vi "run this file.vi"() -> ()   [LabVIEW 2022 SP3]
uses:
  <vilib>/Platform/TimedLoop/XDataNode/timing_clust.ctl
  <vilib>/Platform/TimedLoop/XDataNode/nitl_modes.ctl
  <vilib>/Platform/TimedLoop/XDataNode/wakeup.ctl
  9477/Public/Configure/Setpoint/Configure Setpoint (Percentage).vi
  9477/Public/Data/Setpoint/Read Setpoint (Direct).vi
  Data/Measure/Read Measure (Direct).vi
  <vilib>/Platform/TimedLoop/XDataNode/XDataNode.xnode
  9477/Bronkhorst FLOW-BUS.lvlib
  <vilib>/Platform/TimedLoop/XDataNode/XDNodeRunTimeDep.lvlib
panel:
  out "Numeric":dbl format="%#_13g"
  out "error out 3":errorcluster
  in  "Path":path
  in  "CH4 setpoint percentage":dbl format="%#_13g"
  in  "Air set point percentage":dbl format="%#_13g"
  in  "CO2 set point percentage":dbl format="%#_13g"
  in  "CH4 Node":i32=5
  in  "Air Node":i32=4
  in  "CO2 Node":i32=18
  in  "VISA resource name":refnum<visa-resource-name>="ASRL2::INSTR"
  in  "Stop":bool=TRUE
  out "error out 2":errorcluster
  out "Unit CH4":string
  out "Setpoint Direct (0) CH4":sgl min=0 step=1 format="%#_5g"
  out "Unit Air":string
  out "Setpoint Direct (0) Air":sgl min=0 step=1 format="%#_5g"
  out "Setpoint Direct (0) CO2":sgl min=0 step=1 format="%#_5g"
  out "Unit CO2":string
  # "#This is the visa input resource address, it depends on which kind of the VISA resource user applying."
  # "#The path is the file path the user woyld like to save."
  # "Time"
  # "CO2 flowrate"
  # "Air flowrate"
  # "CH4 flowrate"
  # "# The node is set by the user on the side of Mass Flow Controller itself, swicth the button to the node address you would like to set. \n# The CO2 MFC was used before, and the CO2 node has been set as 18.\n# The Air and CH4 MFC were not used before, the initial setting of node address is 00. \n These two MFC can only show readings when the node addresses are allocated.\n#The expected flowrate of each MFC is set by the percentage, the capacity can be found on the backside of each MFC.\n#Light the STOP button when the suer wants to stop reading."
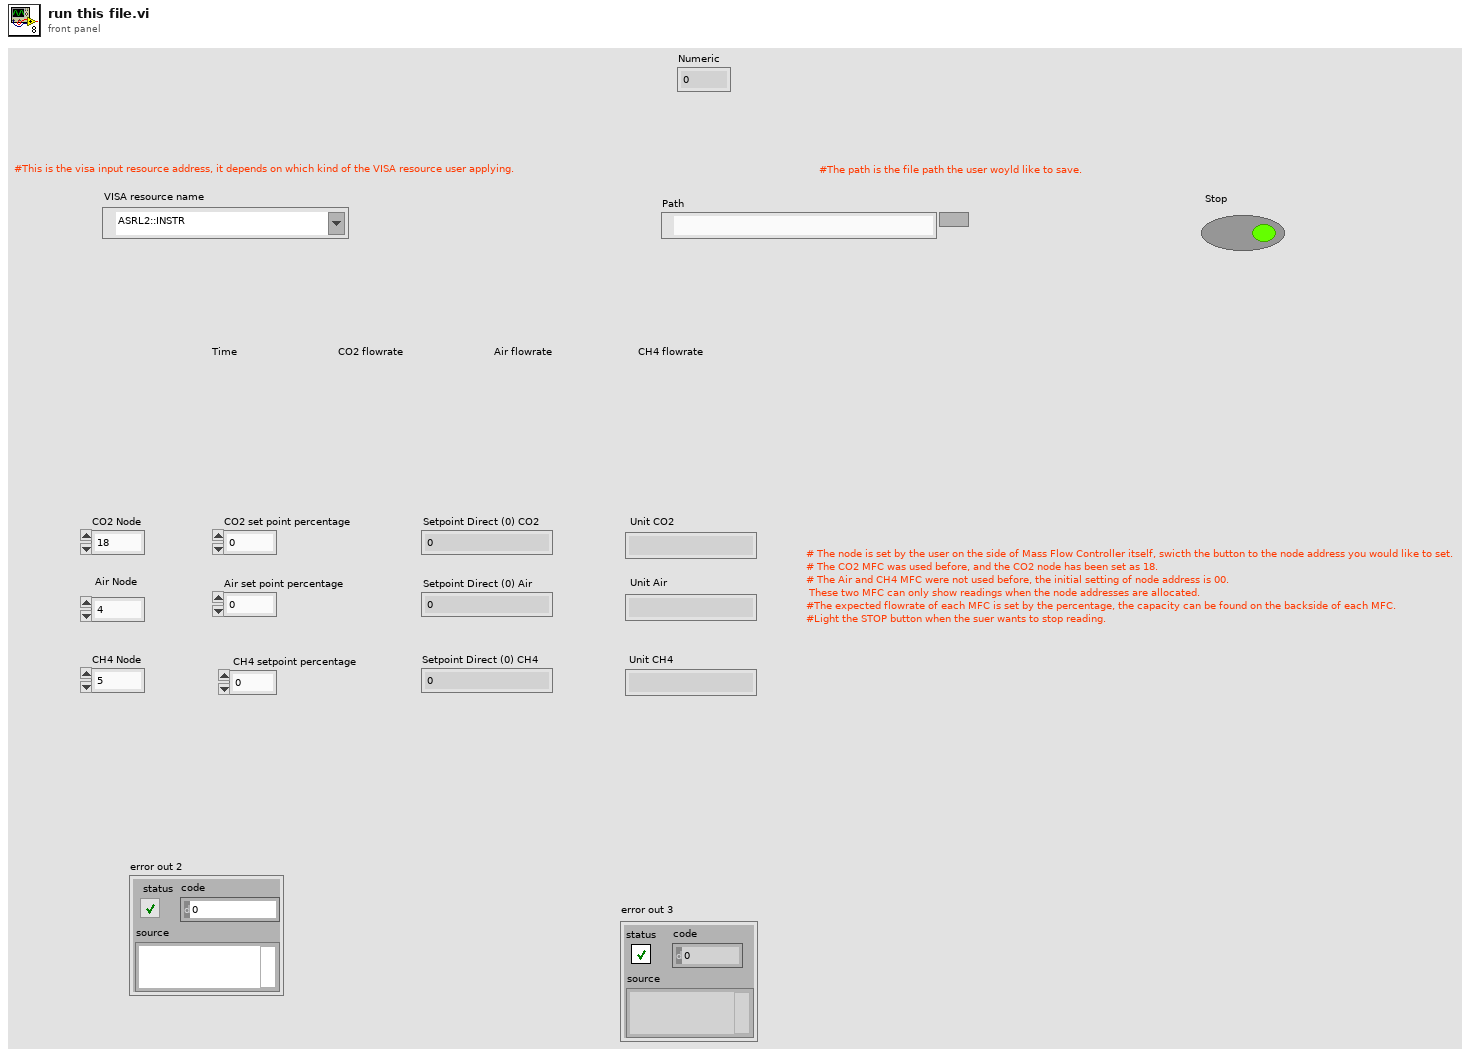
[diagram p1: front panel]
types:
  T1 = enum16{"open", "open or create", "create or replace", "create", "open (read-only)"}
  T2 = typedef "XDNodeRunTimeDep.lvlib/timing_clust.ctl" = cluster{"Expected End [f-1]":u64, "Actual End [f-1]":u64, "Finished Late? [f-1]":bool, "Expected End [i-1]":u64, "Actual End [i-1]":u64, "Finished Late? [i-1]":bool, "Expected Start [i]":u64, "Actual Start [i]":u64, "Expected Start [f]":u64, "Actual Start [f]":u64, "Source Name":string, "Structure Name":string, "Period":i64, "Deadline":i64, "Offset":i64, "Start":i64, "Priority":i32, "Timeout":i32, "Mode":T3, "Wakeup Reason":T4, "Error":errorcluster, "Source Type":string, "Secondary Source Type":string, "Global End Time":u64, "Global Start Time":u64, "Frame Duration":u64, "Iteration Duration":u64, "Assigned CPU":i32, "I/O Scan Engine Mode":u32}
  T3 = typedef "XDNodeRunTimeDep.lvlib/nitl_modes.ctl" = enum32{"No Change", "Process missed periods, maintain original phase", "Discard missed periods, maintain original phase", "Process missed periods, ignore original phase", "Discard missed periods, ignore original phase"}
  T4 = typedef "XDNodeRunTimeDep.lvlib/wakeup.ctl" = enum32{"Normal", "Aborted", "Asynchronous wakeup", "Timing source error", "Timed loop error", "Timeout"}
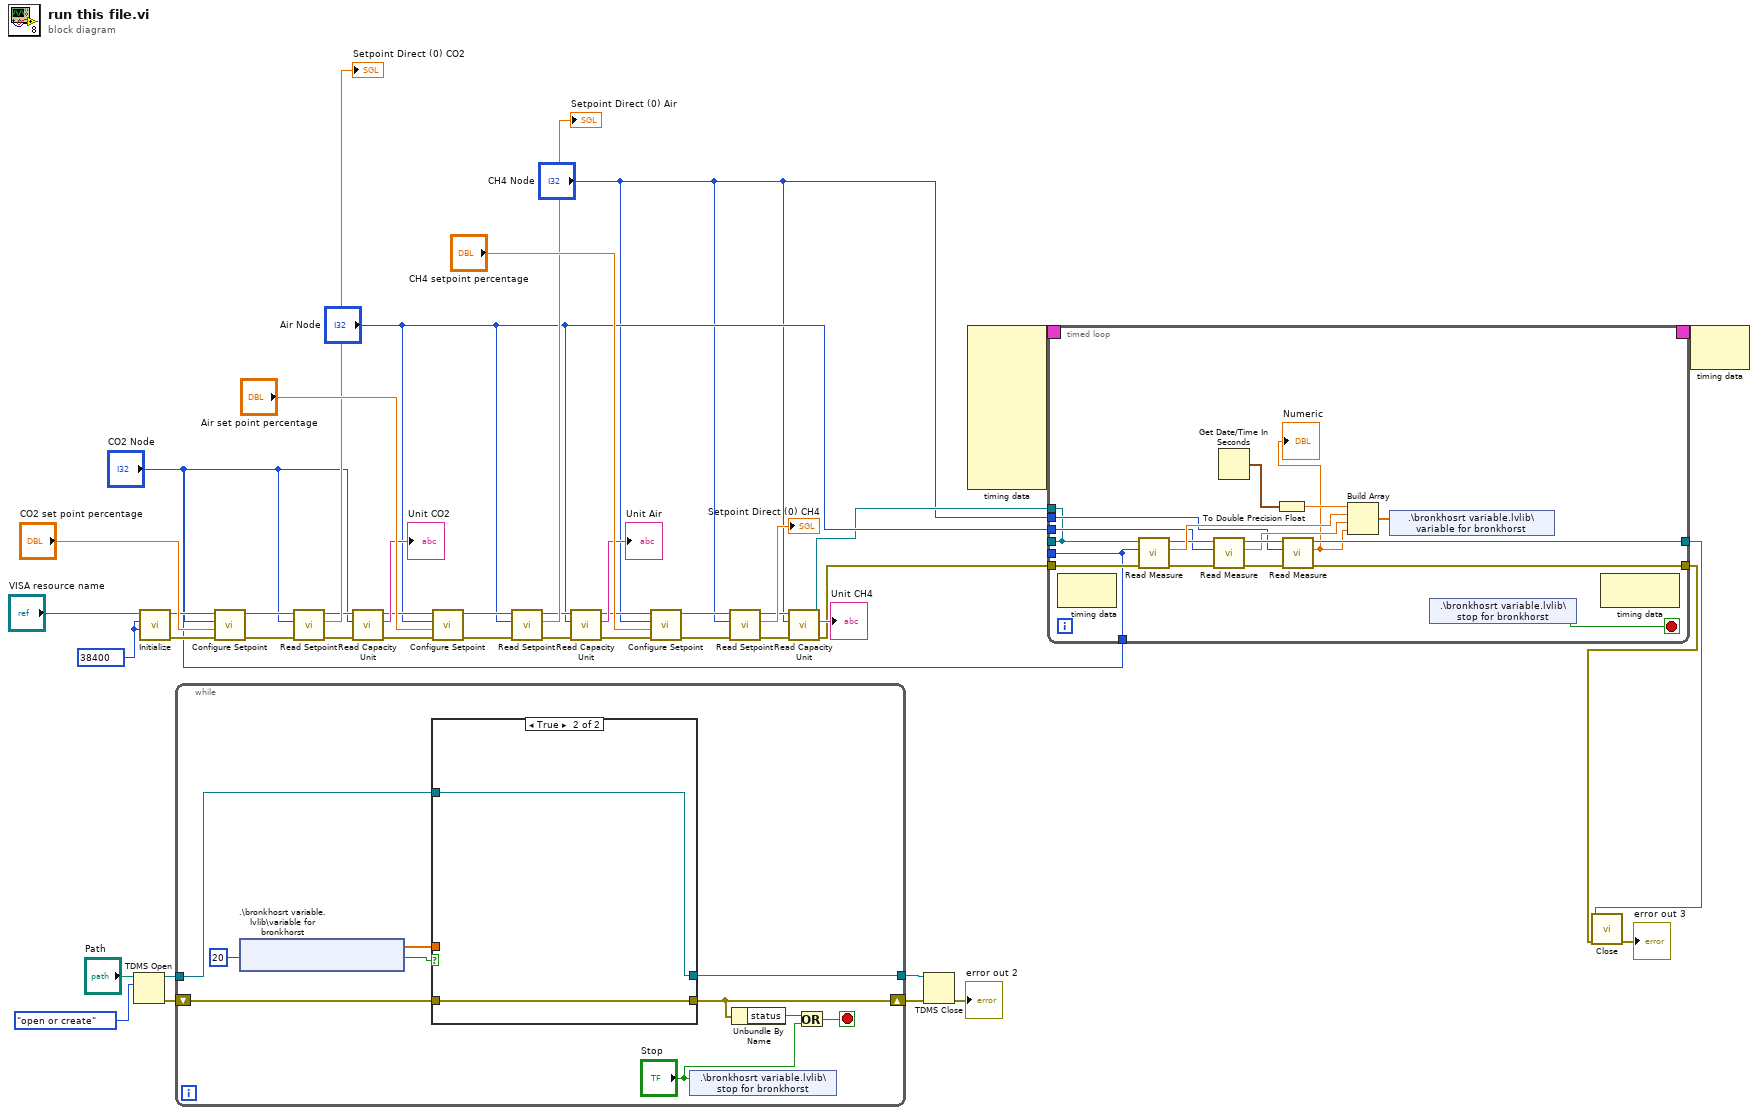
[diagram p0: block diagram]
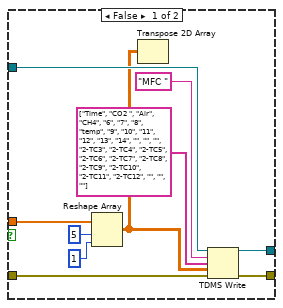
[diagram p2: hidden frame]
diagram:
  w17 = u32 38400 items=["9600"=9600, "19200"=19200, "38400"=38400, "57600"=57600, "115200"=115200, "230400"=230400, "460800"=460800] ("Baud Rate (38400)")
  n1 = TDMS Open(10:T1."open or create" ("operation (0:open)"), 11:"Path") -> (0:w13:errorcluster, 3:w12:refnum<k34>)  [unwired: 5 in]
  n2 = call "Initialize.vi"("Baud Rate (38400)"=w17, "Node (3)"=w17, "VISA resource name"="VISA resource name") -> ("error out"=w37:errorcluster, "VISA resource name out"=w38:refnum<visa-resource-name>)  [unwired: 7 in]
  n3 = while {
    shift-right: [w51] -> w9
    shift-left: w13 -> [w52]
    tunnel: [w49] -> w8
    tunnel: w12 -> [w47]
    stop <- w50 stop-if-true
    n4 = shared-variable ".\\bronkhosrt variable.lvlib\\variable for bronkhorst"(20) -> (w55:dbl[], w53:bool)  [unwired: 1 in, 1 out]
    n5 = case shown="True" w53 {
      tunnel: w52 -> [w64 w68]
      tunnel: w47 -> [w63 w67]
      tunnel: [w62 w67] -> w49
      tunnel: w55 -> [w61 _]
      tunnel: [w57 w68] -> w51
      frame False {
        n6 = Reshape Array(w61, 5, 1) -> (w58:dbl[][])
        n7 = Transpose 2D Array(2D array=w58) -> ()  [unwired: 1 out]
        n8 = TDMS Write(0:w63, 5:"MFC " ("group name in (Untitled)"), 7:string[] ["Time", "CO2 ", "Air", "CH4", "6", "7", "8", "temp", "9", "10", "11", "12", "13", "14", "", "", "", "2-TC3", "2-TC4", "2-TC5", "2-TC6", "2-TC7", "2-TC8", "2-TC9", "2-TC10", "2-TC11", "2-TC12", "", "", ""] ("channel name(s) in (Untitled)"), 9:w58, 11:w64) -> (4:w62:refnum<k34>, 15:w57:errorcluster)  [unwired: 1 in, 2 out]
      }
      frame True {
      }
    }
    n9 = shared-variable ".\\bronkhosrt variable.lvlib\\stop for bronkhorst"("Stop") -> ()  [unwired: 1 in, 1 out]
    n10 = Unbundle By Name(w51) -> ("status"=w54:bool)
    n11 = Or(x=w54, y="Stop") -> (x .or. y?=w50:bool)
  }
  n12 = call-poly "Configure Setpoint.vi"("error in (no error)"=w37, "Setpoint Percentage (0%)"="CO2 set point percentage", "Node (3)"="CO2 Node", "VISA resource name"=w38) -> ("error out"=w33:errorcluster, "VISA resource name out"=w32:refnum<visa-resource-name>)  [unwired: 6 in]
  n13 = call-poly "Read Setpoint.vi"("error in (no error)"=w33, "Node (3)"="CO2 Node", "VISA resource name"=w32) -> ("error out"=w34:errorcluster, "Setpoint Direct"=→"Setpoint Direct (0) CO2":sgl, "VISA resource name out"=w31:refnum<visa-resource-name>)  [unwired: 6 in]
  n14 = call "Read Capacity Unit.vi"("error in (no error)"=w34, "Node (3)"="CO2 Node", "VISA resource name"=w31) -> ("error out"=w25:errorcluster, "Capacity Unit"=→"Unit CO2":string, "VISA resource name out"=w26:refnum<visa-resource-name>)  [unwired: 6 in]
  n15 = call-poly "Configure Setpoint.vi"("error in (no error)"=w25, "Setpoint Percentage (0%)"="Air set point percentage", "Node (3)"="Air Node", "VISA resource name"=w26) -> ("error out"=w29:errorcluster, "VISA resource name out"=w28:refnum<visa-resource-name>)  [unwired: 6 in]
  n16 = call-poly "Read Setpoint.vi"("error in (no error)"=w29, "Node (3)"="Air Node", "VISA resource name"=w28) -> ("error out"=w30:errorcluster, "Setpoint Direct"=→"Setpoint Direct (0) Air":sgl, "VISA resource name out"=w27:refnum<visa-resource-name>)  [unwired: 6 in]
  n17 = call "Read Capacity Unit.vi"("error in (no error)"=w30, "Node (3)"="Air Node", "VISA resource name"=w27) -> ("error out"=w18:errorcluster, "Capacity Unit"=→"Unit Air":string, "VISA resource name out"=w19:refnum<visa-resource-name>)  [unwired: 6 in]
  n18 = call-poly "Configure Setpoint.vi"("error in (no error)"=w18, "Setpoint Percentage (0%)"="CH4 setpoint percentage", "Node (3)"="CH4 Node", "VISA resource name"=w19) -> ("error out"=w22:errorcluster, "VISA resource name out"=w21:refnum<visa-resource-name>)  [unwired: 6 in]
  n19 = call-poly "Read Setpoint.vi"("error in (no error)"=w22, "Node (3)"="CH4 Node", "VISA resource name"=w21) -> ("error out"=w23:errorcluster, "Setpoint Direct"=→"Setpoint Direct (0) CH4":sgl, "VISA resource name out"=w20:refnum<visa-resource-name>)  [unwired: 6 in]
  n20 = call "Read Capacity Unit.vi"("error in (no error)"=w23, "Node (3)"="CH4 Node", "VISA resource name"=w20) -> ("error out"=w7:errorcluster, "Capacity Unit"=→"Unit CH4":string, "VISA resource name out"=w2:refnum<visa-resource-name>)  [unwired: 6 in]
  n21 = TDMS Close(8:w9, 11:w8) -> (0:→"error out 2":errorcluster)  [unwired: 1 out]
  n22 = node-c288() -> (w15:T2)  [unwired: 9 in]
  n23 = timed-loop {
    timing: w15 -> [_]
    timing-out: [_] -> w14
    tunnel: [w71] -> _
    tunnel: "Air Node" -> [w76]
    tunnel: "CH4 Node" -> [w75]
    tunnel: [w74] -> w5
    tunnel: [w73] -> w6
    tunnel: w7 -> [w72]
    tunnel: [w70] -> _
    tunnel: "CO2 Node" -> [w71]
    tunnel: w2 -> [w70]
    stop <- w79 stop-if-true
    n24 = node-c288() -> ()  [unwired: 1 in, 1 out]
    n25 = call-poly "Read Measure.vi"("error in (no error)"=w72, "Node (3)"=w71, "VISA resource name"=w70) -> ("error out"=w83:errorcluster, "Measure Direct"=w86:sgl, "VISA resource name out"=w85:refnum<visa-resource-name>)  [unwired: 6 in]
    n26 = call-poly "Read Measure.vi"("error in (no error)"=w83, "Node (3)"=w76, "VISA resource name"=w85) -> ("error out"=w82:errorcluster, "Measure Direct"=w77:sgl, "VISA resource name out"=w84:refnum<visa-resource-name>)  [unwired: 6 in]
    n27 = Get Date/Time In Seconds() -> (seconds since 1Jan1904=w78:timestamp)
    n28 = To Double Precision Float(number=w78) -> (double precision float=w80:dbl)
    n29 = call-poly "Read Measure.vi"("error in (no error)"=w82, "Node (3)"=w75, "VISA resource name"=w84) -> ("error out"=w73:errorcluster, "Measure Direct"=w69:sgl, "VISA resource name out"=w74:refnum<visa-resource-name>)  [unwired: 6 in]
    "Numeric" <- w69
    n30 = Build Array(w80, w86, w77, w69) -> (w81:dbl[])
    n31 = shared-variable ".\\bronkhosrt variable.lvlib\\variable for bronkhorst"(w81) -> ()  [unwired: 1 in, 1 out]
    n32 = shared-variable ".\\bronkhosrt variable.lvlib\\stop for bronkhorst"() -> (w79:bool)  [unwired: 1 in, 1 out]
    n33 = node-c288() -> ()  [unwired: 1 in, 1 out]
  }
  n34 = call "Close.vi"("error in (no error)"=w6, "VISA resource name"=w5) -> ("error out"=→"error out 3":errorcluster)  [unwired: 9 in]
  n35 = node-c288(w14) -> ()  [unwired: 1 out]
